vi "Register Events.vi"(8 "error in (no error)":errorcluster, 11 "2DArrayManager in":refnum<class "2DArrayManager.lvclass">) -> (0 "error out":errorcluster, 3 "2DArrayManager out":refnum<class "2DArrayManager.lvclass">)   [LabVIEW 2020, in "OOPanel.lvlib" / "2DArrayManager.lvclass"]
uses:
  2DArrayManager.lvclass
  2DArrayManager.lvclass/2DArrayManager.ctl
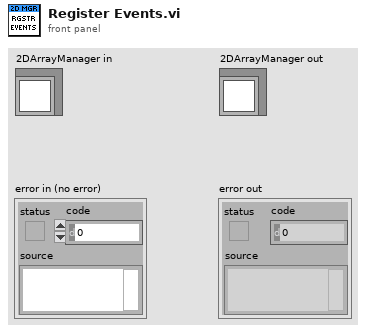
[diagram p1: front panel]
types:
  T1 = typedef "OOPanel.lvlib/2DArrayManager.lvclass/Events.ctl" = cluster{"Stop":refnum<user-event>, "Update":refnum<user-event>, "Set BG":refnum<user-event>, "Scroll":refnum<user-event>, "Highlight":refnum<user-event>, "Synced Scroll":refnum<user-event>}
  T2 = typedef "OOPanel.lvlib/2DArrayManager.lvclass/Event Reg Ref.ctl" = cluster{"Last Update Ticks ms":u32, "Event Reg":refnum<event-registration>}
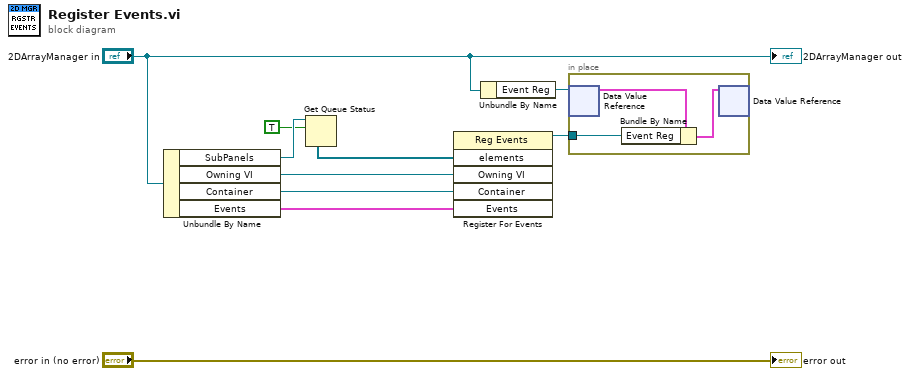
[diagram p0: block diagram]
diagram:
  n1 = Unbundle By Name("2DArrayManager in") -> ("SubPanels"=w3:refnum<queue>, "Owning VI"=w7:refnum<vi>, "Container"=w4:refnum<vi>, "Events"=w6:T1)
  n2 = Get Queue Status(queue=w3, return elements? (F)=TRUE) -> (elements=w1:refnum<vi>[])  [unwired: 1 in, 7 out]
  n3 = register-events(w1, w7, w4, w6) -> (reference out=w5:refnum<event-registration>)  [unwired: 2 in, 1 out]
  n4 = Unbundle By Name("2DArrayManager in") -> ("Event Reg"=w9:refnum<data-value>)
  n5 = in-place {
    in-place-border: w5 -> [w11]
    n6 = in-place-dvr #1(w9) -> (w13:T2)  [unwired: 1 out]
    n7 = Bundle By Name(cluster=w13, "Event Reg"=w11) -> (w12:T2)
    n8 = in-place-dvr #1(w12) -> ()  [unwired: 2 out]
  }
  "error out" <- "error in (no error)"
  "2DArrayManager out" <- "2DArrayManager in"
